vi "SetupWindow.vi"(8 "error in (no error)":errorcluster) -> (0 "error out":errorcluster)   [LabVIEW 2015]
doc: "Setup Windows display the setup data"
uses:
  global_variables.vi
panel:
  in  "Export Folder":path
  in  "Source Folder":path
  in  "Save button":bool
  in  "Data Source":enum32{"Folder", "Database"}(radio)
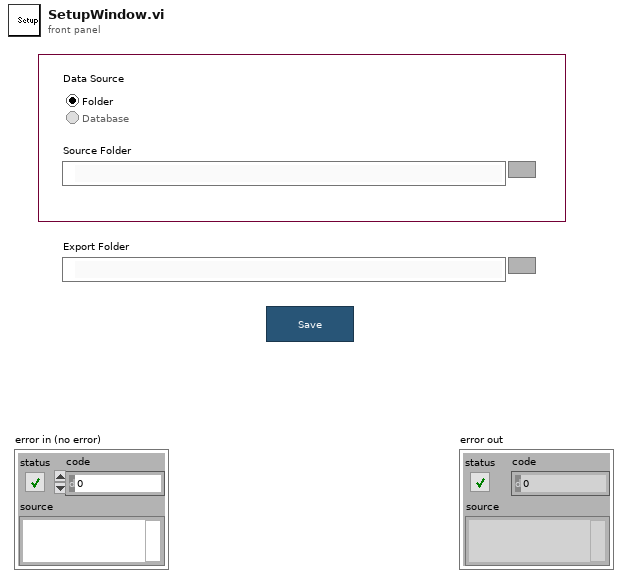
[diagram p1: front panel]
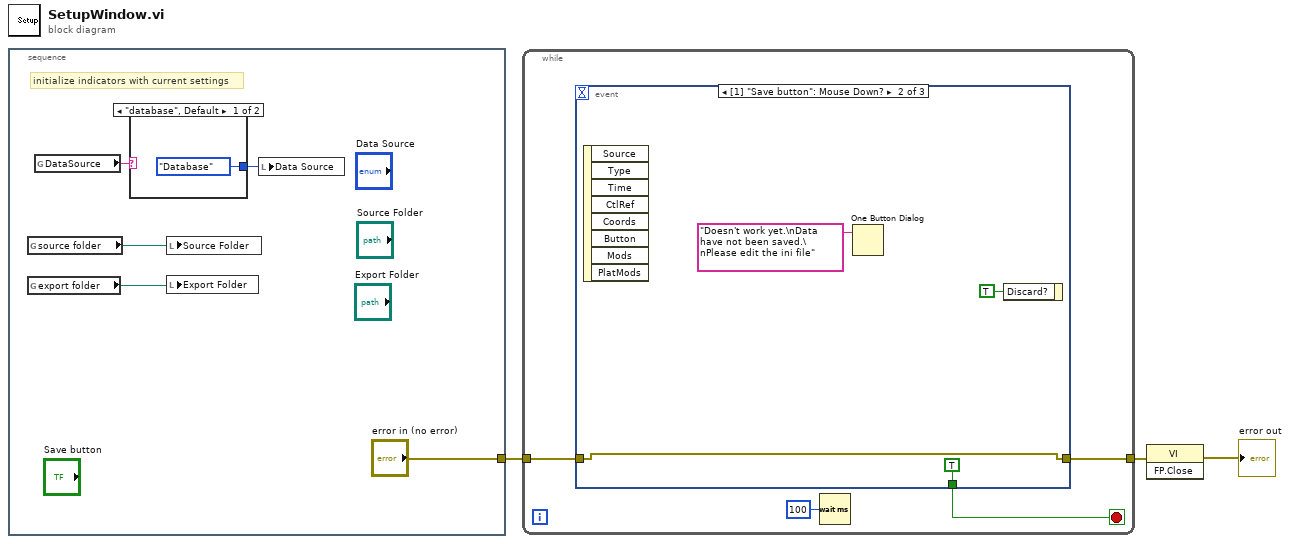
[diagram p0: block diagram]
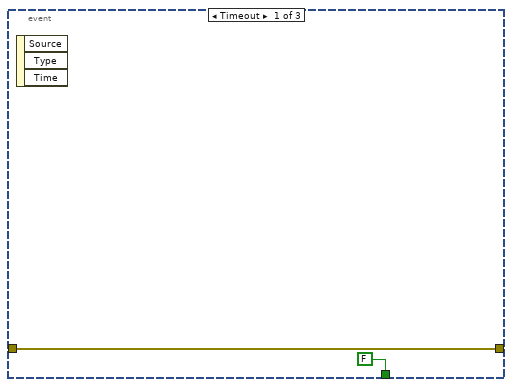
[diagram p2: hidden frame]
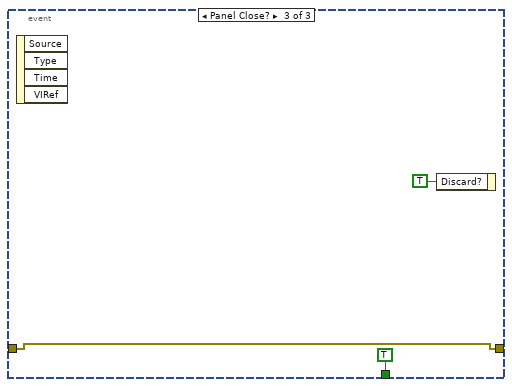
[diagram p3: hidden frame]
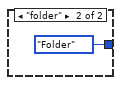
[diagram p4: hidden frame]
diagram:
  n1 = stacked-sequence {
    tunnel: ["error in (no error)"] -> w3
    frame #0 {
      # "initialize indicators with current settings"
      n2 = global read "global_variables.vi" "source folder"() -> (w6:path)
      n3 = global read "global_variables.vi" "export folder"() -> (w5:path)
      n4 = global read "global_variables.vi" "DataSource"() -> (w8:string)
      n5 = case shown="\"database\", Default" w8 {
        tunnel: [enum32{"Folder", "Database"}."Database" ("Data Source") enum32{"Folder", "Database"}."Folder" ("Data Source")] -> w7
        frame "database", Default {
        }
        frame "folder" {
        }
      }
      n6 = local write "Source Folder"(w6) -> ()
      n7 = local write "Export Folder"(w5) -> ()
      n8 = local write "Data Source"(w7) -> ()
    }
  }
  n9 = while {
    tunnel: w3 -> [w14]
    tunnel: [w13] -> w2
    stop <- w12 stop-if-true
    n10 = event shown="[1] \"Save button\": Mouse Down?" {
      selector: _ -> [_ _ _]
      dyn-events: _ -> [_ _ _]
      timeout: _ -> [_ _ _]
      tunnel: w14 -> [w16 w18 w21]
      tunnel: [w16 w18 w21] -> w13
      tunnel: [FALSE TRUE TRUE] -> w12
      event Timeout {
        n11 = event-data() -> ()  [unwired: 1 in, 3 out]
      }
      event "Save button": Mouse Down? {
        n12 = event-data() -> ()  [unwired: 1 in, 8 out]
        n13 = One Button Dialog(message="Doesn't work yet.\nData have not been saved.\nPlease edit the ini file") -> ()  [unwired: 1 in, 1 out]
        n14 = event-data("Discard?"=TRUE) -> ()  [unwired: 1 in, 1 out]
      }
      event Panel Close? {
        n15 = event-data() -> ()  [unwired: 1 in, 4 out]
        n16 = event-data("Discard?"=TRUE) -> ()  [unwired: 1 in, 1 out]
      }
    }
    n17 = Wait (ms)(milliseconds to wait=u32 100) -> ()  [unwired: 1 out]
  }
  n18 = invoke class="VI" method="FP.Close"(error in=w2) -> (error out=→"error out":errorcluster)  [unwired: 2 in, 2 out]
